vi "Status Pressure Limits.vi"(5 "Retry Attempts (0)":i32 min=0, 8 "error in (no error)":errorcluster, 11 "VISA resource name":refnum<visa-resource-name>) -> (0 "error out":errorcluster, 1 "Lower Pressure Limit":dbl, 2 "Upper Pressure Limit":dbl, 3 "VISA resource name out":refnum<visa-resource-name>)   [LabVIEW 2020, in "ChromTech Series III Pump.lvlib"]
doc: "Query pump for upper and lower pressure limits."
uses:
  <instrlib>/RxnRover/ChromtechSeriesIIIDriver/ChromTech Series III Pump.lvlib
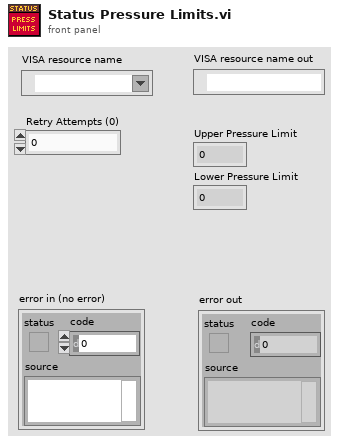
[diagram p1: front panel]
types:
  T1 = cluster{"Flow rate":dbl, "Upper Pressure Limit":dbl, "Lower Pressure Limit":dbl, "Pressure Units":string, "Running?":bool, "Pressure Board Present?":bool, "Macro Pump Head?":bool}
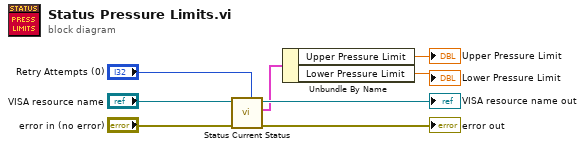
[diagram p0: block diagram]
diagram:
  n1 = call <instrlib>:"Status Current Status.vi"("Retry Attempts (0)"="Retry Attempts (0)", "error in (no error)"="error in (no error)", "VISA resource name"="VISA resource name") -> ("error out"=→"error out":errorcluster, "Status Cluster"=w4:T1, "VISA resource name out"=→"VISA resource name out":refnum<visa-resource-name>)  [unwired: 6 in]
  n2 = Unbundle By Name(w4) -> ("Upper Pressure Limit"=→"Upper Pressure Limit":dbl, "Lower Pressure Limit"=→"Lower Pressure Limit":dbl)
